vi "Vector to Euler angle.vi"(0 "A Vector":sgl[](array[numeric])) -> (1 "alpha":sgl, 2 "beta":sgl)   [LabVIEW 2018]
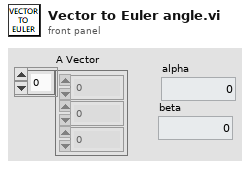
[diagram p1: front panel]
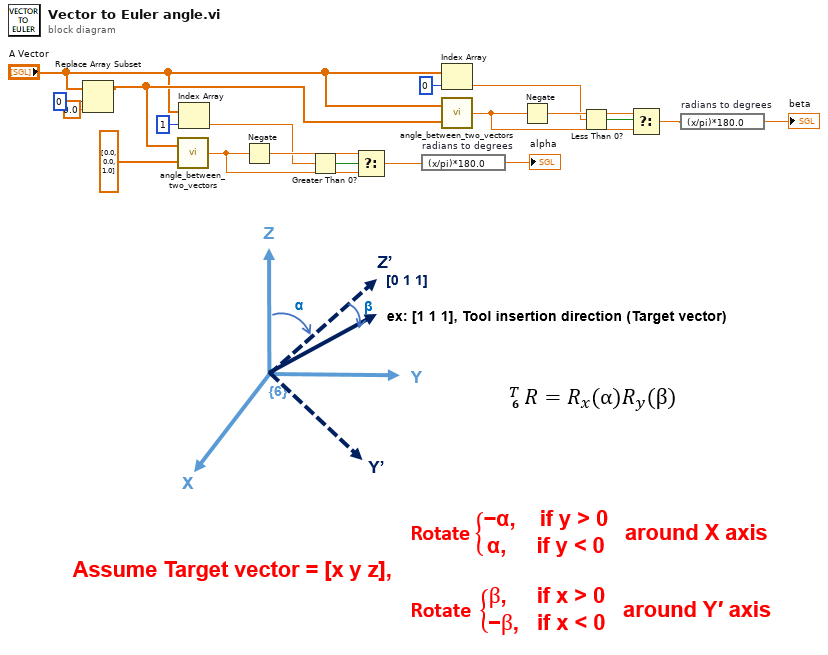
[diagram p0: block diagram]
diagram:
  n1 = Replace Array Subset(array="A Vector", new element=0.0 ("new element/subarray"), index=0) -> (w14:sgl[])
  n2 = call "angle_between_two_vectors.vi"("B Vector"=dbl[] [0.0, 0.0, 1.0], "A Vector"=w14) -> ("degree"=w16:dbl)
  n3 = Index Array(array="A Vector", index=1) -> (element=w6:sgl)
  n4 = Negate(x=w16) -> (-x=w15:dbl)
  n5 = Greater Than 0?(x=w6) -> (x > 0?=w5:bool)
  n6 = Select(t=w15, s=w5, f=w16) -> (s? t:f=w9:dbl)
  n7 = expression code="(x/pi)*180.0" "radians to degrees"(w9) -> (→"alpha":dbl)
  n8 = Index Array(array="A Vector", index=0) -> (element=w2:sgl)
  n9 = call "angle_between_two_vectors.vi"("B Vector"=w14, "A Vector"="A Vector") -> ("degree"=w13:dbl)
  n10 = Negate(x=w13) -> (-x=w10:dbl)
  n11 = Less Than 0?(x=w2) -> (x < 0?=w1:bool)
  n12 = Select(t=w10, s=w1, f=w13) -> (s? t:f=w12:dbl)
  n13 = expression code="(x/pi)*180.0" "radians to degrees"(w12) -> (→"beta":dbl)
